vi "Waypoint Controller Main.vi"(11 "Instance Details":T1) -> ()   [LabVIEW 2014]
uses:
  Aircraft Information/Sub VI/Get Aircraft Waypoints.vi
  Controls/MAVLINK Mav Frame.ctl
  Controls/Mission Planning Controls/MAVLINK Mission Item.ctl
  Commands/Mission Planning/MISSION_ACK SubVI/INVALID SEQUENCE.vi
  Commands/Mission Planning/MISSION_ACK SubVI/ACCEPTED.vi
  FGV/Methods/Set Waypoint Transfer Status.vi
  FGV/Methods/Get Waypoint Transfer Status.vi
  Application Support/Stop Button/SubVI/Get Stop Button Status.vi
  Settings File/SubVI/Load Overlord Mode.vi
  Telemetry/Controls/Telemetry Connection Type.ctl
  Ground Station to Aircraft Coms/SubVI/Hardware Driver/Controls/Coms Driver Interface.ctl
  Ground Station to Aircraft Coms/SubVI/Aircraft Data Router/Controls/Known Aircraft.ctl
  <vilib>/httpClient/ClientHandle.ctl
  <vilib>/httpClient/LabVIEWHTTPClient.lvlib
panel:
  out "concatenated string":string
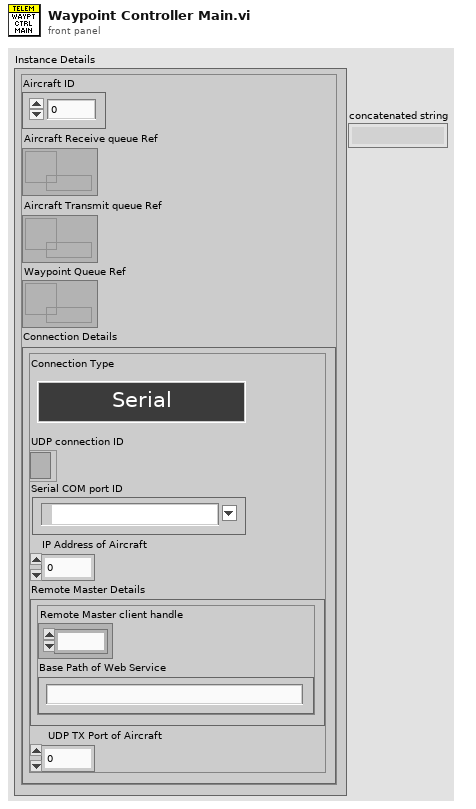
[diagram p1: front panel]
types:
  T1 = typedef "Known Aircraft.ctl" = cluster{"Aircraft ID":u8, "Aircraft Receive queue Ref":refnum<queue>, "Aircraft Transmit queue Ref":refnum<queue>, "Waypoint Queue Ref":refnum<queue>, "Connection Details":T2}
  T2 = typedef "Coms Driver Interface.ctl" = cluster{"Connection Type":T3, "UDP connection ID":refnum<k16>, "Serial COM port ID":refnum<visa-resource-name>, "IP Address of Aircraft":u32, "Remote Master Details":cluster{"Remote Master client handle":T4, "Base Path of Web Service":string}, "UDP TX Port of Aircraft":u16}
  T3 = typedef "Telemetry Connection Type.ctl" = enum16{"Serial", "UDP", "Remote Master"}
  T4 = typedef "LabVIEWHTTPClient.lvlib/ClientHandle.ctl" = refnum<k1>
  T5 = typedef "MAVLINK Mission Item.ctl" = cluster{"target_system":u8, "target_component":u8, "sequence":u16, "frame":T6, "command":u16, "current":bool, "autocontinue":bool, "param1":sgl, "param2":sgl, "param3":sgl, "param4":sgl, "Lat":sgl, "Lon":sgl, "Altitude (m)":sgl}
  T6 = typedef "MAVLINK Mav Frame.ctl" = enum8{"GLOBAL", "LOCAL NED", "MISSION", "GLOBAL RELATIVE ALT", "LOCAL ENU", "GLOBAL INT", "GLOBAL RELATIVE ALT INT", "LOCAL OFFSET NED", "BODY NED", "BODY OFFSET NED", "GLOBAL TERRAIN ALT", "GLOBAL TERRAIN ALT INT"}
  T7 = typedef "Waypoint Transfer Status.ctl" = cluster{"Upload Complete":bool, "Transfer Progress (Upload)":dbl, "Download Complete":bool, "Transfer Progress (Download)":dbl}
  T8 = typedef "MAVLink Packet.ctl" = cluster{"Payload Length":u8, "Packet Sequence":u8, "System ID":u8, "Component ID":u8, "Message ID":u8, "Data":string, "Checksum":u16}
  T9 = typedef "MAVLink Mission Ack.ctl" = cluster{"type":u8, "Description":string}
  T10 = cluster{"target_system":u8, "target_component":u8, "sequence":u16, "frame":T6, "command":u16, "current":bool, "autocontinue":bool, "param1":sgl, "param2":sgl, "param3":sgl, "param4":sgl, "x":sgl, "y":sgl, "z":sgl}[]
  T11 = cluster{"target_system":u8, "target_component":u8, "sequence":u16, "frame":T6, "command":u16, "current":bool, "autocontinue":bool, "param1":sgl, "param2":sgl, "param3":sgl, "param4":sgl, "x":sgl, "y":sgl, "z":sgl}
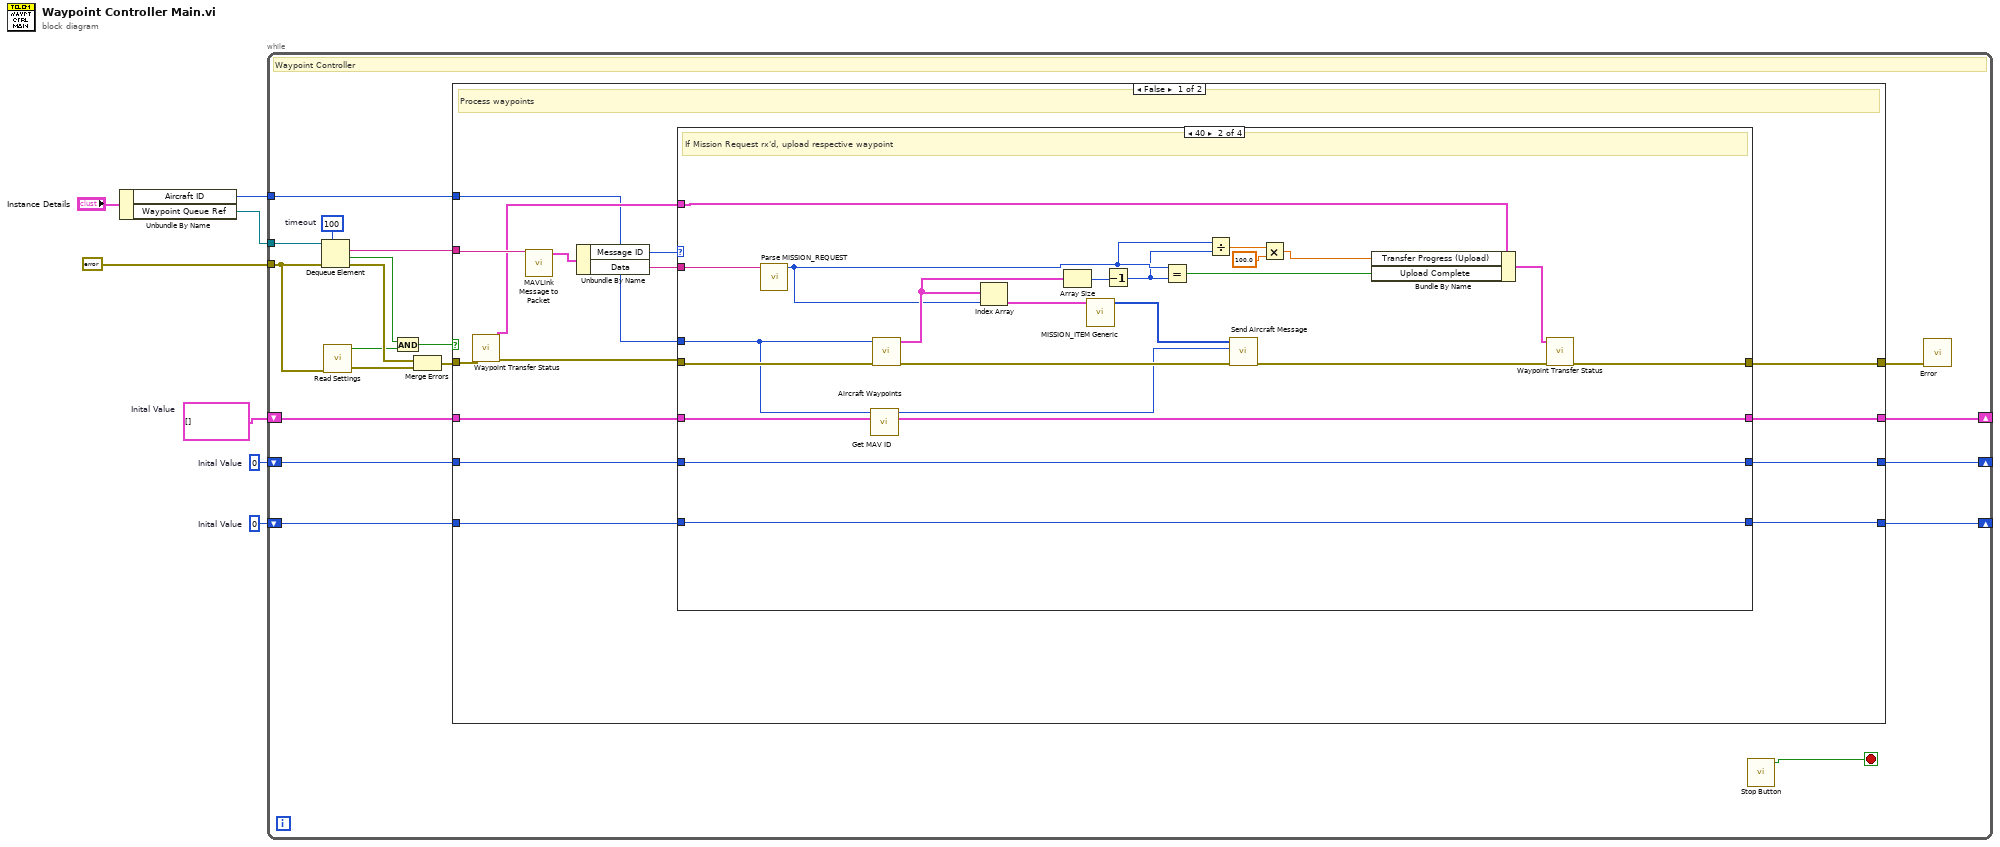
[diagram p0: block diagram]
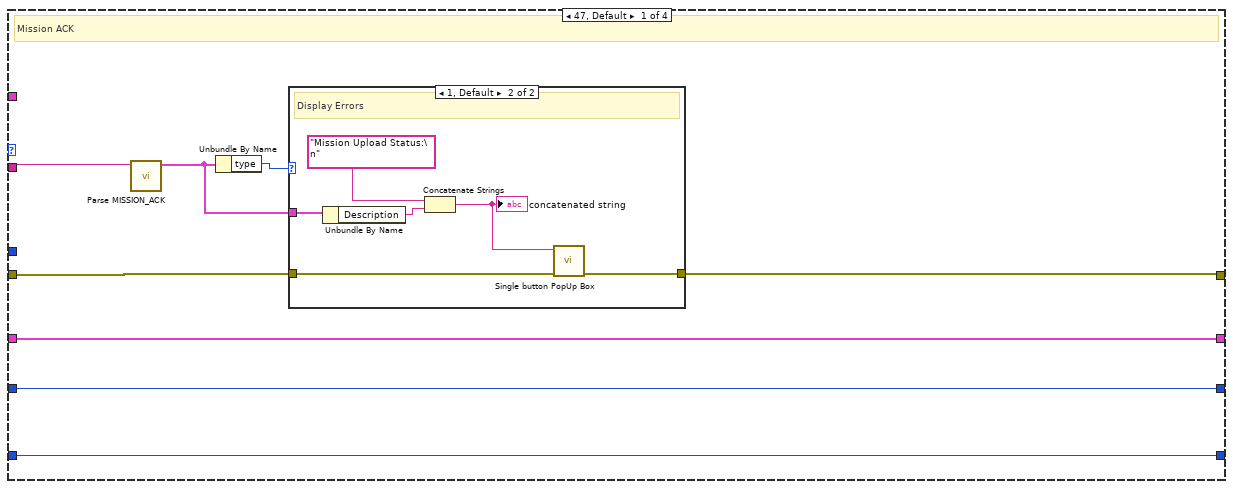
[diagram p2: hidden frame]
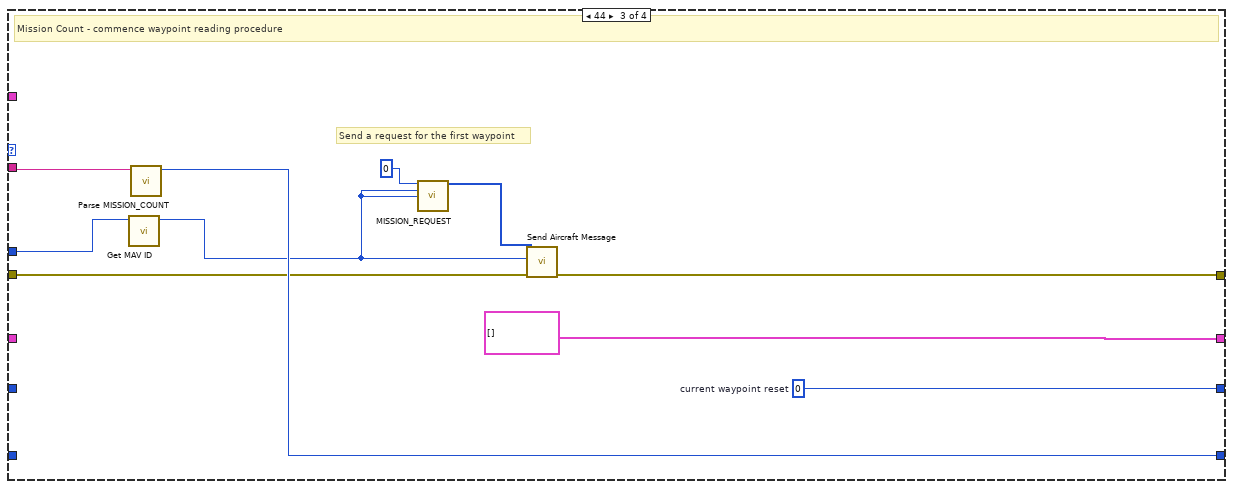
[diagram p4: hidden frame]
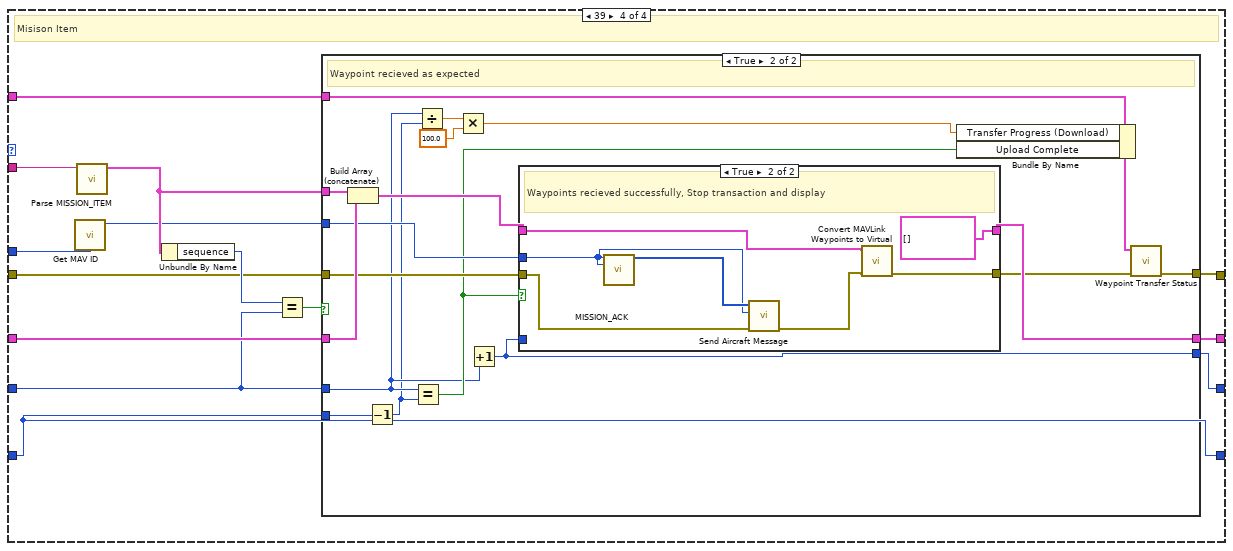
[diagram p5: hidden frame]
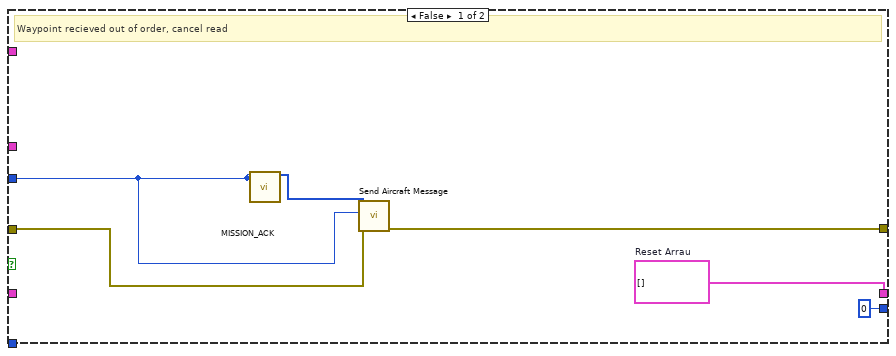
[diagram p6: hidden frame]
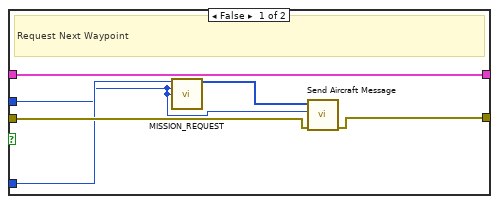
[diagram p7: hidden frame]
diagram:
  w1 = u16 0  # Inital Value
  w2 = u16 0  # Inital Value
  w3 = T5[] []  # Inital Value
  n1 = Unbundle By Name("Instance Details") -> ("Aircraft ID"=w5:u8, "Waypoint Queue Ref"=w6:refnum<queue>)
  n2 = while {
    tunnel: w6 -> [w24]
    tunnel: w5 -> [w23]
    tunnel: errorcluster {"status"=FALSE, "code"=0, "source"=""} ("Error In") -> [w11]
    shift-right: [w21] -> _
    shift-left: w3 -> [w20]
    shift-right: [w19] -> _
    shift-left: w2 -> [w18]
    shift-right: [w17] -> _
    shift-left: w1 -> [w16]
    stop <- w22 stop-if-true
    w26 = 100  # timeout
    # "Waypoint Controller"
    n3 = Dequeue Element(queue=w24, timeout in ms (-1)=w26, error in (no error)=w11) -> (element=w25:string, timed out?=w9:bool, error out=w13:errorcluster)  [unwired: 1 out]
    n4 = call-poly "Read Settings.vi"("Error In"=w11) -> ("error out"=w14:errorcluster, "Master (T)"=w10:bool)  [unwired: 9 in]
    n5 = And(x=w9, y=w10) -> (x .and. y?=w8:bool)
    n6 = Merge Errors(w13, w14) -> (w12:errorcluster)
    n7 = case shown="False" w8 {
      tunnel: w25 -> [w41 _]
      tunnel: w12 -> [w36 w143]
      tunnel: [w37 w143] -> w15
      tunnel: w23 -> [w33 _]
      tunnel: [w32 w142] -> w21
      tunnel: w20 -> [w31 w142]
      tunnel: [w29 w141] -> w19
      tunnel: w18 -> [w30 w141]
      tunnel: [w28 w140] -> w17
      tunnel: w16 -> [w27 w140]
      frame False {
        # "Process waypoints"
        n8 = call-poly "Waypoint Transfer Status.vi"("Error In"=w36) -> ("Error Out"=w35:errorcluster, "Waypoint Transfer Status Out"=w34:T7)  [unwired: 9 in]
        n9 = call "MAVLink Message to Packet.vi"("Message"=w41) -> ("Packet"=w40:T8)  [unwired: 9 in, 1 out]
        n10 = Unbundle By Name(w40) -> ("Message ID"=w39:u8, "Data"=w38:string)
        n11 = case shown="40" w39 {
          tunnel: w38 -> [w49 w78 w88 w102]
          tunnel: w35 -> [w42 w77 w85 w98]
          tunnel: w33 -> [_ w75 w86 w91]
          tunnel: [w43 w66 w84 w92] -> w37
          tunnel: w27 -> [w48 w71 _ w99]
          tunnel: [w48 w71 w87 w99] -> w28
          tunnel: w31 -> [w46 w69 _ w96]
          tunnel: [w46 w69 T5[] [] w95] -> w32
          tunnel: w30 -> [w47 w70 _ w94]
          tunnel: [w47 w70 w79 w93] -> w29
          tunnel: w34 -> [_ w64 _ w89]
          frame 47, Default {
            # "Mission ACK"
            n12 = call "Parse MISSION_ACK.vi"("Data"=w49) -> ("Mission Acknowledge"=w45:T9)  [unwired: 10 in]
            n13 = Unbundle By Name(w45) -> ("type"=w44:u8)
            n14 = case shown="1, Default" w44 {
              tunnel: w45 -> [_ w54]
              tunnel: w42 -> [w50 w52]
              tunnel: [w50 w51] -> w43
              frame 0 {
                # "No Upload error"
              }
              frame 1, Default {
                # "Display Errors"
                n15 = Unbundle By Name(w54) -> ("Description"=w55:string)
                n16 = Concatenate Strings("Mission Upload Status:\n" ("string"), w55) -> (w53:string)
                "concatenated string" <- w53
                n17 = call "Single button PopUp Box.vi"("Error In"=w52, "Input Message"=w53) -> ("Error Out"=w51:errorcluster)  [unwired: 8 in, 1 out]
              }
            }
          }
          frame 40 {
            # "If Mission Request rx'd, upload respective waypoint"
            n18 = call "Parse MISSION_REQUEST.vi"("Data"=w78) -> ("Waypoint Number"=w61:u16)  [unwired: 10 in]
            n19 = call "Get MAV ID.vi"("Aircraft Index"=w75) -> ("Aircraft ID"=w72:u8)  [unwired: 9 in, 1 out]
            n20 = call-poly "Aircraft Waypoints.vi"("Error In"=w77, "Aircraft ID"=w75) -> ("Error Out"=w73:errorcluster, "Waypoints Out"=w68:T10)  [unwired: 8 in]
            n21 = Index Array(array=w68, index=w61) -> (element=w76:T11)
            n22 = Array Size(array=w68) -> (size(s)=w67:i32)
            n23 = call "MISSION_ITEM Generic.vi"("MISSION_ITEM"=w76) -> ("MAVLink Message"=w74:u8[])  [unwired: 10 in]
            n24 = Decrement(x=w67) -> (x-1=w60:i32)
            n25 = Equal?(x=w61, y=w60) -> (x = y?=w63:bool)
            n26 = Divide(x=w61, y=w60) -> (x/y=w59:dbl)
            n27 = call "Send Aircraft Message.vi"("error in (no error)"=w73, "Aircraft ID"=w72, "MAVLink Message"=w74) -> ("error out"=w65:errorcluster)  [unwired: 8 in]
            n28 = Multiply(x=w59, y=100.0) -> (x*y=w57:dbl)
            n29 = Bundle By Name(cluster=w64, "Transfer Progress (Upload)"=w57, "Upload Complete"=w63) -> (w62:T7)
            n30 = call-poly "Waypoint Transfer Status.vi"("Error In"=w65, "Waypoint Transfer Status In"=w62) -> ("Error Out"=w66:errorcluster)  [unwired: 9 in]
          }
          frame 44 {
            w79 = u16 0  # current waypoint reset
            # "Send a request for the first waypoint"
            # "Mission Count - commence waypoint reading procedure"
            n31 = call "Get MAV ID.vi"("Aircraft Index"=w86) -> ("Aircraft ID"=w83:u8)  [unwired: 9 in, 1 out]
            n32 = call "Parse MISSION_COUNT.vi"("Data"=w88) -> ("Number of Mission Items"=w87:u16)  [unwired: 10 in]
            n33 = call "MISSION_REQUEST.vi"("sequence"=u16 0, "target_system"=w83, "target_component"=w83) -> ("MAVLink Message"=w82:u8[])  [unwired: 12 in]
            n34 = call "Send Aircraft Message.vi"("error in (no error)"=w85, "Aircraft ID"=w83, "MAVLink Message"=w82) -> ("error out"=w84:errorcluster)  [unwired: 8 in]
          }
          frame 39 {
            # "Misison Item"
            n35 = call "Get MAV ID.vi"("Aircraft Index"=w91) -> ("Aircraft ID"=w90:u8)  [unwired: 9 in, 1 out]
            n36 = call "Parse MISSION_ITEM.vi"("Data"=w102) -> ("Mission Item"=w97:T5)  [unwired: 10 in]
            n37 = Unbundle By Name(w97) -> ("sequence"=w101:u16)
            n38 = Equal?(x=w101, y=w94) -> (x = y?=w100:bool)
            n39 = case shown="True" w100 {
              tunnel: w99 -> [_ w124]
              tunnel: w98 -> [w105 w120]
              tunnel: w97 -> [_ w126]
              tunnel: w96 -> [_ w125]
              tunnel: [w104 w122] -> w95
              tunnel: w94 -> [_ w113]
              tunnel: [u16 0 w119] -> w93
              tunnel: [w108 w118] -> w92
              tunnel: w90 -> [w106 w121]
              tunnel: w89 -> [_ w116]
              frame False {
                w104 = T5[] []  # Reset Arrau
                # "Waypoint recieved out of order, cancel read"
                n40 = call-poly "MISSION_ACK.vi"("target_system"=w106, "target_component"=w106) -> ("MAVLink Message"=w107:u8[])  [unwired: 13 in]
                n41 = call "Send Aircraft Message.vi"("error in (no error)"=w105, "Aircraft ID"=w106, "MAVLink Message"=w107) -> ("error out"=w108:errorcluster)  [unwired: 8 in]
              }
              frame True {
                # "Waypoint recieved as expected"
                n42 = Build Array (concatenate)(w126, w125) -> (w123:T5[])
                n43 = Decrement(x=w124) -> (x-1=w112:u16)
                n44 = Equal?(x=w113, y=w112) -> (x = y?=w114:bool)
                n45 = Divide(x=w113, y=w112) -> (x/y=w111:dbl)
                n46 = Multiply(x=w111, y=100.0) -> (x*y=w109:dbl)
                n47 = Increment(x=w113) -> (x+1=w119:u16)
                n48 = case shown="True" w114 {
                  tunnel: w123 -> [w132 w133]
                  tunnel: [w132 T5[] []] -> w122
                  tunnel: w121 -> [w127 w138]
                  tunnel: w120 -> [w130 w137]
                  tunnel: [w131 w135] -> w117
                  tunnel: w119 -> [w129 _]
                  frame False {
                    # "Request Next Waypoint"
                    n49 = call "MISSION_REQUEST.vi"("sequence"=w129, "target_system"=w127, "target_component"=w127) -> ("MAVLink Message"=w128:u8[])  [unwired: 12 in]
                    n50 = call "Send Aircraft Message.vi"("error in (no error)"=w130, "Aircraft ID"=w127, "MAVLink Message"=w128) -> ("error out"=w131:errorcluster)  [unwired: 8 in]
                  }
                  frame True {
                    # "Waypoints recieved successfully, Stop transaction and display"
                    n51 = call-poly "MISSION_ACK.vi"("target_system"=w138, "target_component"=w138) -> ("MAVLink Message"=w139:u8[])  [unwired: 13 in]
                    n52 = call "Send Aircraft Message.vi"("error in (no error)"=w137, "Aircraft ID"=w138, "MAVLink Message"=w139) -> ("error out"=w134:errorcluster)  [unwired: 8 in]
                    n53 = call "Convert MAVLink Waypoints to Virtual.vi"("Error In"=w134, "Mavlink Waypoints"=w133) -> ("Error Out"=w135:errorcluster)  [unwired: 9 in]
                  }
                }
                n54 = Bundle By Name(cluster=w116, "Transfer Progress (Download)"=w109, "Upload Complete"=w114) -> (w115:T7)
                n55 = call-poly "Waypoint Transfer Status.vi"("Error In"=w117, "Waypoint Transfer Status In"=w115) -> ("Error Out"=w118:errorcluster)  [unwired: 9 in]
              }
            }
          }
        }
      }
      frame True {
        # "Timed out. Do nothing"
      }
    }
    n56 = call-poly "Stop Button.vi"() -> ("Stop ButtonOut"=w22:bool)  [unwired: 10 in, 1 out]
    n57 = call "Error.vi"("Error In"=w15) -> ()  [unwired: 10 in, 1 out]
  }
